vi "Controller - Fire Position Change.vi"(8 "error in (no error)":errorcluster, 10 "Position":T1, 11 "View Model":T2) -> (0 "error out":errorcluster, 3 "View Model":T2)   [LabVIEW 2017]
doc: "Generate User Event = Position Change"
uses:
  View Model/Controls/View Model.ctl
  View Model/Controls/Shared Model.ctl
  Error/Controls/Error Model.ctl
  Error/Controls/Error Event.ctl
  Error/Controls/Error Type.ctl
  Configuration/Controls/Config DB Model.ctl
  Configuration/Controls/Config DB Command.ctl
  Configuration/Controls/Config DB Record.ctl
  Controls/Controller Model.ctl
  Controls/Elevator Location.ctl
  Controls/Elevator Direction Event.ctl
  Controls/Elevator Direction.ctl
  Controls/Elevator CMD Event.ctl
  Controls/Elevator Commands.ctl
  Controls/Elevator Overhead.ctl
  Controls/Elevator State.ctl
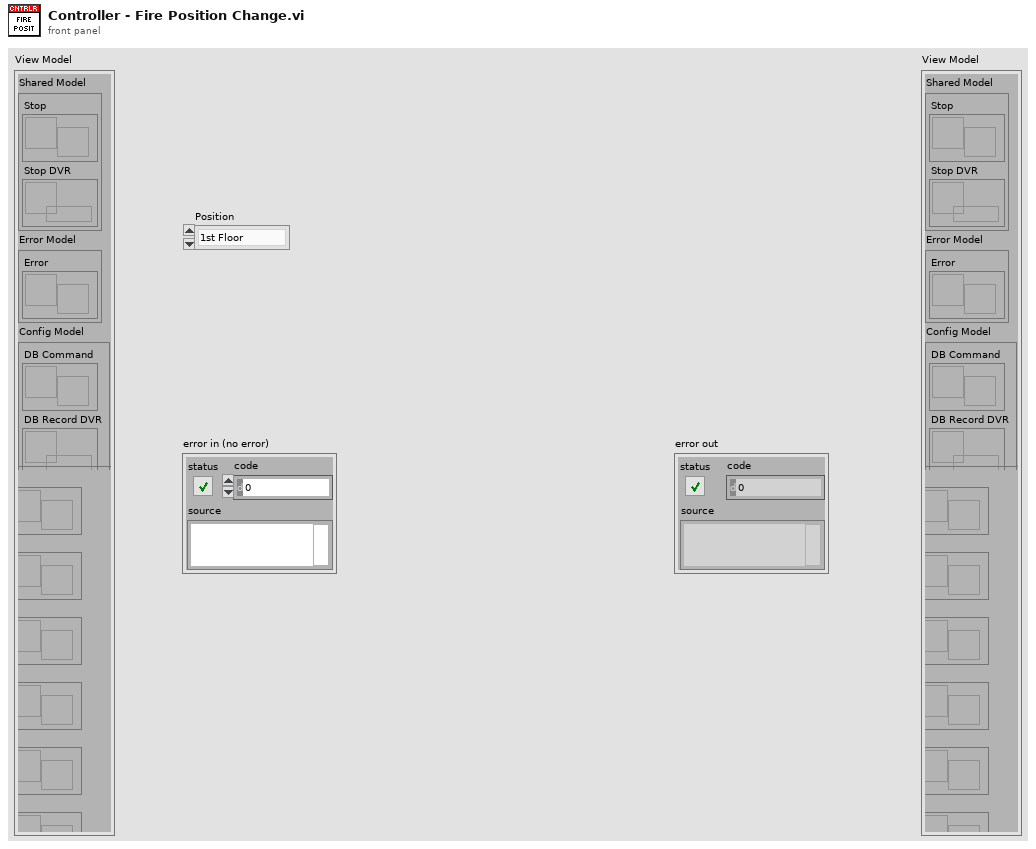
[diagram p1: front panel]
types:
  T1 = typedef "Elevator Location.ctl" = enum16{"1st Floor", "2nd Floor", "3rd Floor", "4th Floor"}
  T2 = typedef "View Model.ctl" = cluster{"Shared Model":T3, "Error Model":T4, "Config Model":T5, "Controller Model":T6}
  T3 = typedef "Shared Model.ctl" = cluster{"Stop":refnum<user-event>, "Stop DVR":refnum<data-value>}
  T4 = typedef "Error Model.ctl" = cluster{"Error":refnum<user-event>}
  T5 = typedef "Config DB Model.ctl" = cluster{"DB Command":refnum<user-event>, "DB Record DVR":refnum<data-value>}
  T6 = typedef "Controller Model.ctl" = cluster{"Go to Floor":refnum<user-event>, "Emergency":refnum<user-event>, "Open/Close Door":refnum<user-event>, "Move To":refnum<user-event>, "Position Change":refnum<user-event>, "Elevator CMD Event":refnum<user-event>, "Overhead DVR":refnum<data-value>, "Motion Event":refnum<user-event>}
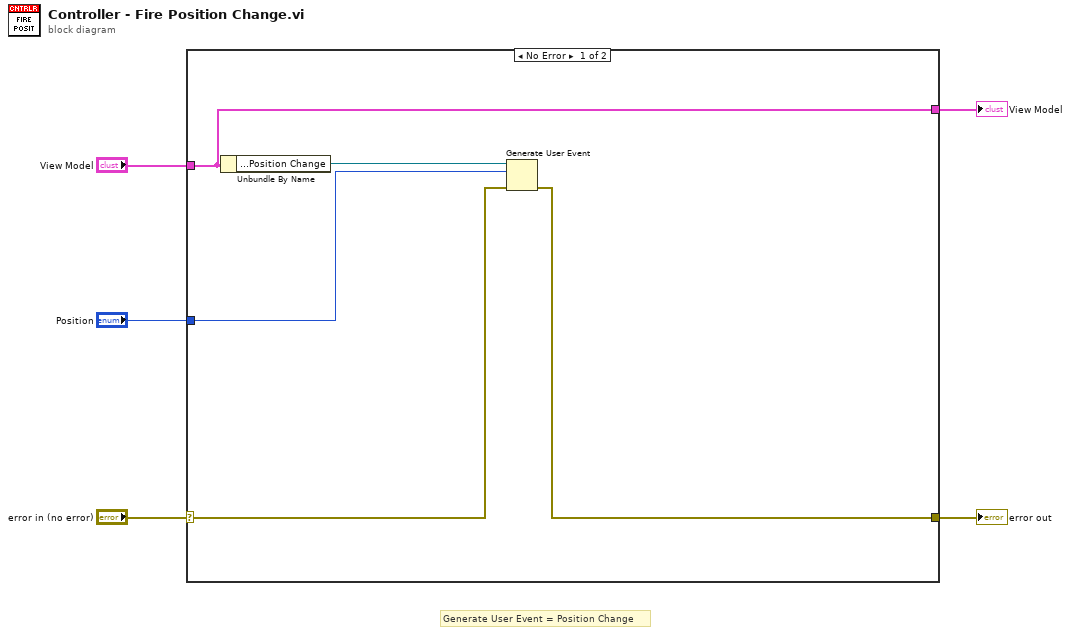
[diagram p0: block diagram]
diagram:
  # "Generate User Event = Position Change"
  n1 = case shown="No Error" "error in (no error)" {
    selector: "error in (no error)" -> [w9 w11]
    tunnel: "View Model" -> [w7 w12]
    tunnel: [w7 w12] -> w3
    tunnel: [w8 w11] -> w2
    tunnel: "Position" -> [w6 _]
    frame No Error {
      n2 = Unbundle By Name(w7) -> ("Controller Model.Position Change"=w10:refnum<user-event>)
      n3 = Generate User Event(user event=w10, event data cluster=w6, error in=w9) -> (error out=w8:errorcluster)  [unwired: 1 in, 1 out]
    }
    frame Error {
    }
  }
  "error out" <- w2
  "View Model" <- w3
